vi "PipelineDuty.vi"(8 "error in (no error)":errorcluster, 10 "DataExchange":T1, 11 "Device in":refnum<class "Device.lvclass">) -> (0 "error out":errorcluster, 2 "DataExchange 2":T1, 3 "Device out":refnum<class "Device.lvclass">)   [LabVIEW 2020, in "Device.lvlib" / "Device.lvclass"]
uses:
  Device.lvclass
  DataExchange.ctl
  <vilib>/vision/Image Controls.llb/IMAQ Image.ctl
  GenericActor/GenericActor/GenericActor.lvclass
  Interface/DataListener/DataListener.lvclass
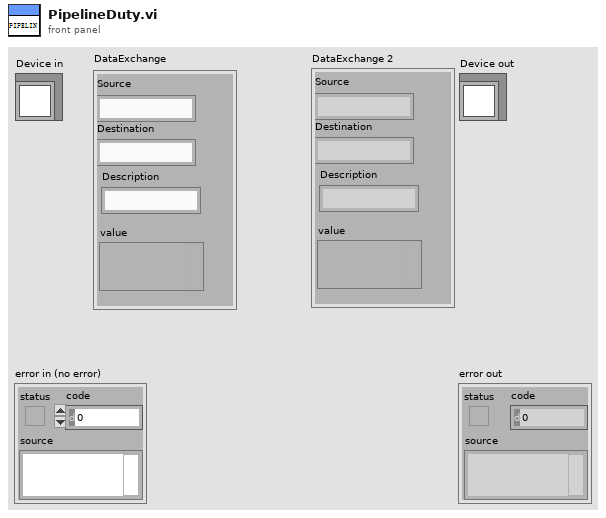
[diagram p1: front panel]
types:
  T1 = typedef "DataListener.lvclass/DataExchange.ctl" = cluster{"Source":string, "Destination":string, "Description":string, "value":variant}
  T2 = typedef "IMAQ Image.ctl" = refnum<image>
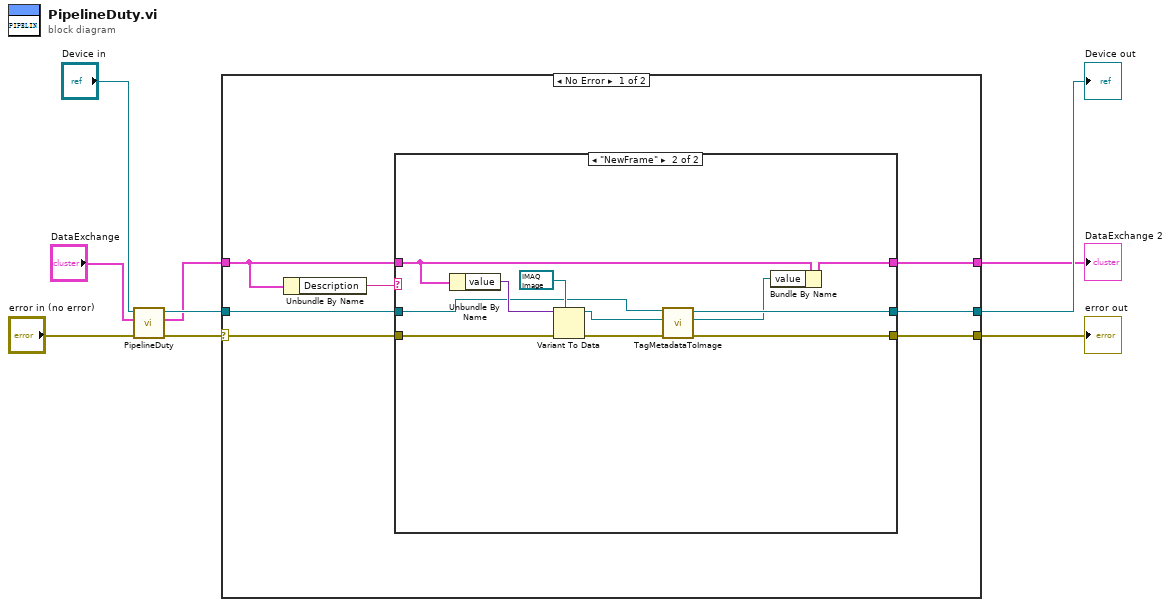
[diagram p0: block diagram]
diagram:
  n1 = call-parent "PipelineDuty.vi"("error in (no error)"="error in (no error)", "DataExchange"="DataExchange", "GRMActor in"="Device in") -> ("error out"=w6:errorcluster, "DataExchange 2"=w1:T1, "GRMActor out"=w4:refnum<class "Device.lvclass">)  [unwired: 6 in]
  n2 = case shown="No Error" w6 {
    selector: w6 -> [w16 w31]
    tunnel: [w15 w31] -> w5
    tunnel: w4 -> [w14 w32]
    tunnel: [w13 w32] -> w3
    tunnel: [w12 w33] -> w2
    tunnel: w1 -> [w11 w33]
    frame No Error {
      n3 = Unbundle By Name(w11) -> ("Description"=w10:string)
      n4 = case shown="\"NewFrame\"" w10 {
        tunnel: w16 -> [w17 w30]
        tunnel: [w17 w29] -> w15
        tunnel: w14 -> [w18 w21]
        tunnel: [w18 w28] -> w13
        tunnel: w11 -> [w19 w26]
        tunnel: [w19 w27] -> w12
        frame Default {
        }
        frame "NewFrame" {
          n5 = Unbundle By Name(w26) -> ("value"=w24:variant)
          n6 = Variant To Data(error in=w30, type=T2 refnum ("Image In"), Variant=w24) -> (data=w22:T2, error out=w25:errorcluster)
          n7 = call-dynamic "TagMetadataToImage.vi"("error in (no error)"=w25, "Image In"=w22, "Device in"=w21) -> ("error out"=w29:errorcluster, "Image Out"=w20:T2, "Device out"=w28:refnum<class "Device.lvclass">)  [unwired: 6 in]
          n8 = Bundle By Name(cluster=w26, "value"=w20) -> (w27:T1)
        }
      }
    }
    frame Error {
    }
  }
  "error out" <- w5
  "Device out" <- w3
  "DataExchange 2" <- w2
